vi "Read Array of ccd.vi"(11 "CCD monitor in":refnum<class "CCD monitor.lvclass">) -> (2 "Array of ccd":refnum<class "CCD.lvclass">[](array[class]), 3 "CCD monitor out":refnum<class "CCD monitor.lvclass">)   [LabVIEW 2016, in "CCD monitor.lvlib" / "CCD monitor.lvclass"]
uses:
  <userlib>/Common Components/Hardware/Abstract System/Monitor/CCD monitor.lvclass
  <userlib>/Common Components/Hardware/CCD/CCD/CCD.lvclass
  <userlib>/Common Components/Hardware/Abstract System/Monitor/CCD monitor.lvclass/CCD monitor.ctl
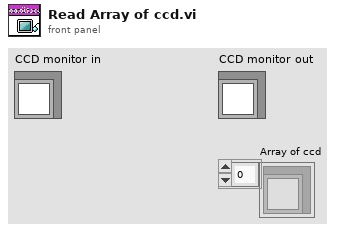
[diagram p1: front panel]
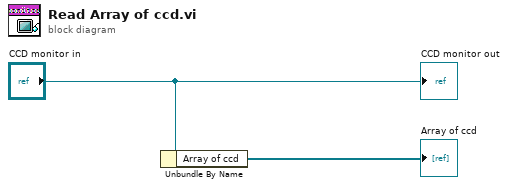
[diagram p0: block diagram]
diagram:
  n1 = Unbundle By Name("CCD monitor in") -> ("Array of ccd"=→"Array of ccd":refnum<class "CCD.lvclass">[])
  "CCD monitor out" <- "CCD monitor in"
